vi "ReadSettings.vi"() -> (1 "Settings":T1)   [LabVIEW 2015]
uses:
  <vilib>/Utility/sysdir.llb/System Directory Type.ctl
  <vilib>/registry/registry.llb/Registry RtKey.ctl
  <vilib>/registry/registry.llb/Registry SAM.ctl
  Ctrls/YesOrNo.ctl
  <vilib>/Utility/config.llb/Read Key (U32).vi
  <vilib>/registry/registry.llb/Read Registry Value Simple STR.vi
  <vilib>/Utility/config.llb/Write Key (U32).vi
  <vilib>/Utility/config.llb/Read Key (Boolean).vi
  <vilib>/Utility/config.llb/Write Key (Boolean).vi
  <vilib>/Utility/config.llb/NI_LVConfig.lvlib
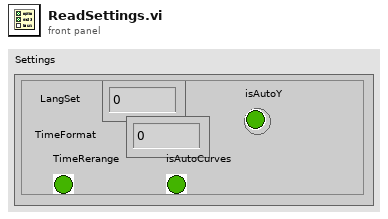
[diagram p1: front panel]
types:
  T1 = cluster{"LangSet":u32, "TimeFormat":u16, "TimeRerange":bool, "isAutoCurves":bool, "isAutoY":bool}
  T2 = typedef "System Directory Type.ctl" = i32
  T3 = typedef "NI_LVConfig.lvlib/Config Data RefNum.ctl" = refnum<k1>
  T4 = typedef "Registry SAM.ctl" = enum32{"KEY_QUERY_VALUE", "KEY_SET_VALUE", "KEY_CREATE_SUB_KEY", "KEY_ENUMERATE_SUB_KEYS", "KEY_NOTIFY", "KEY_CREATE_LINK", "KEY_READ", "KEY_WRITE", "KEY_ALL_ACCESS", "KEY_READ | KEY_WRITE"}
  T5 = typedef "Registry RtKey.ctl" = enum32{"HKEY_CLASSES_ROOT", "HKEY_CURRENT_USER", "HKEY_LOCAL_MACHINE", "HKEY_USERS", "HKEY_PERFORMANCE_DATA", "HKEY_CURRENT_CONFIG", "HKEY_DYN_DATA"}
  T6 = typedef "Registry refnum.ctl" = refnum<k1>
  T7 = typedef "YesOrNo.ctl" = bool
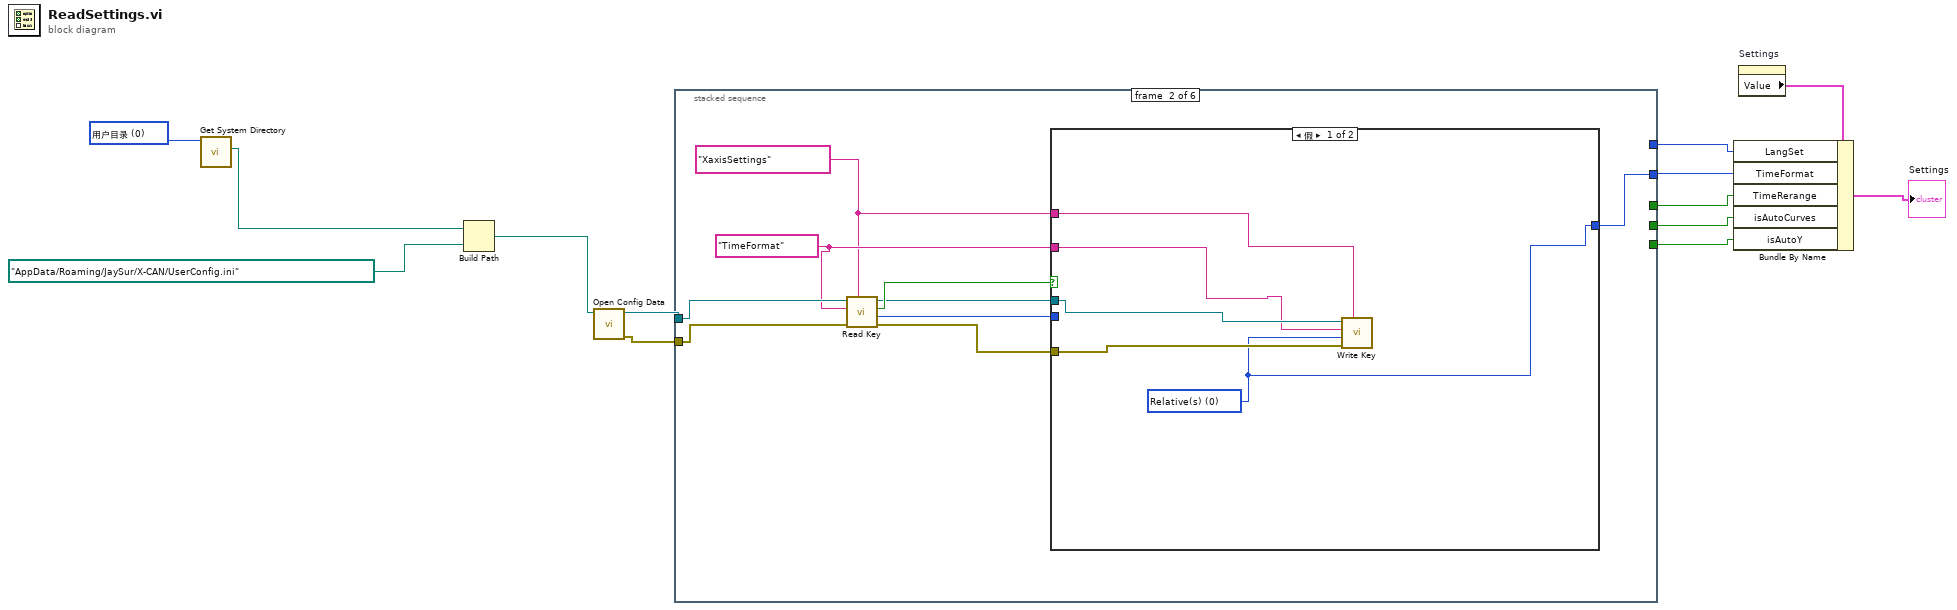
[diagram p0: block diagram]
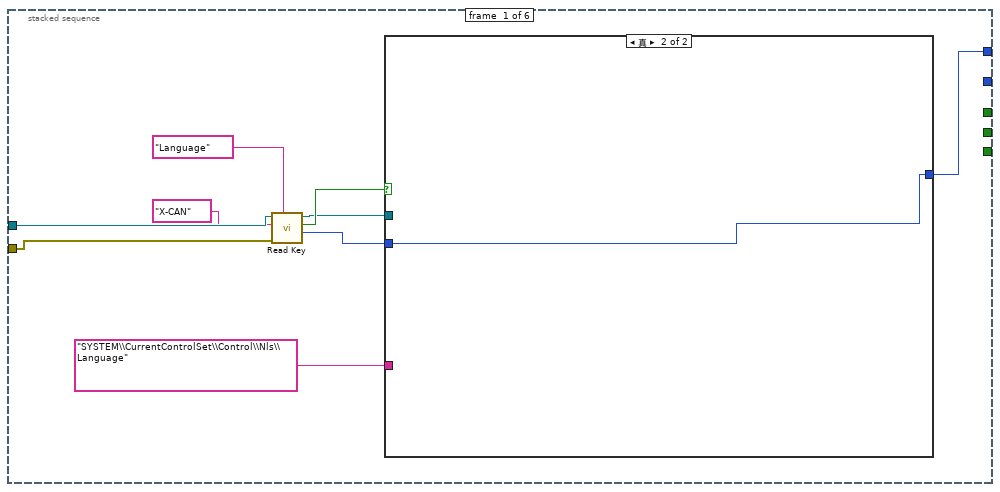
[diagram p2: hidden frame]
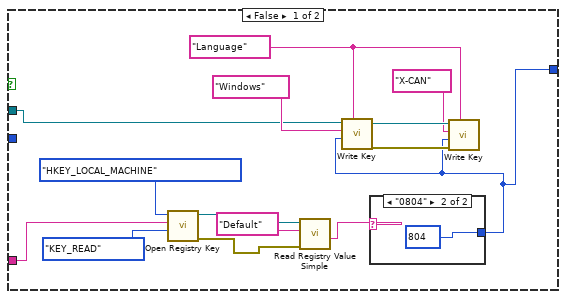
[diagram p3: hidden frame]
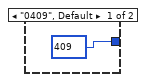
[diagram p4: hidden frame]
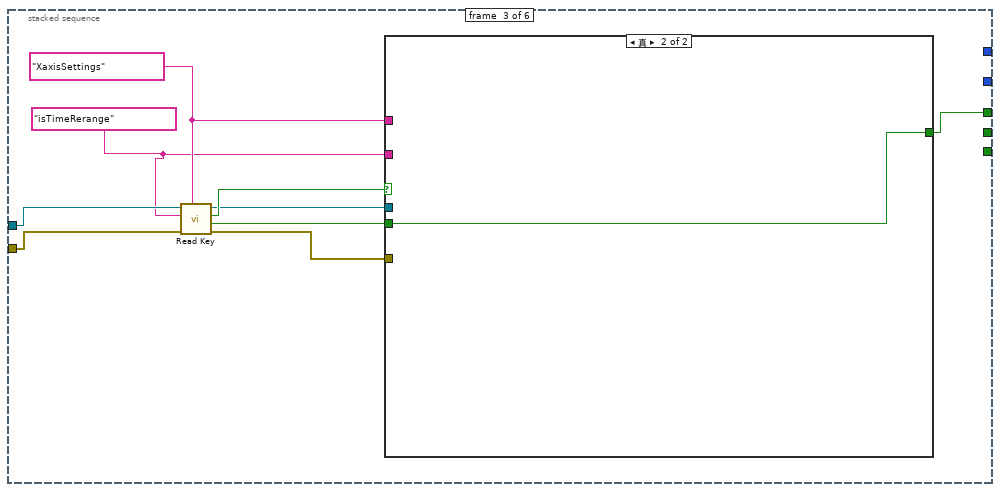
[diagram p6: hidden frame]
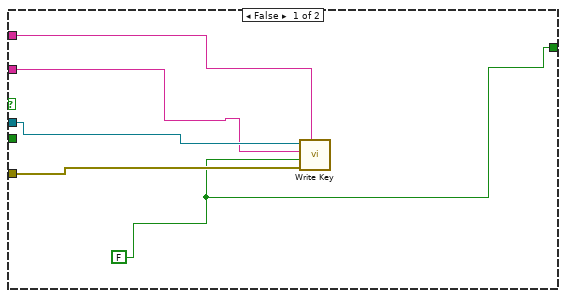
[diagram p7: hidden frame]
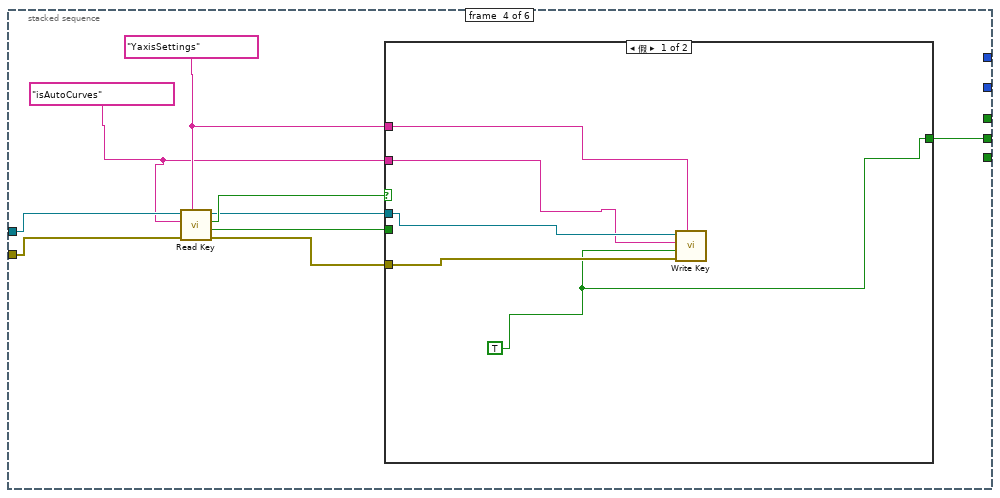
[diagram p8: hidden frame]
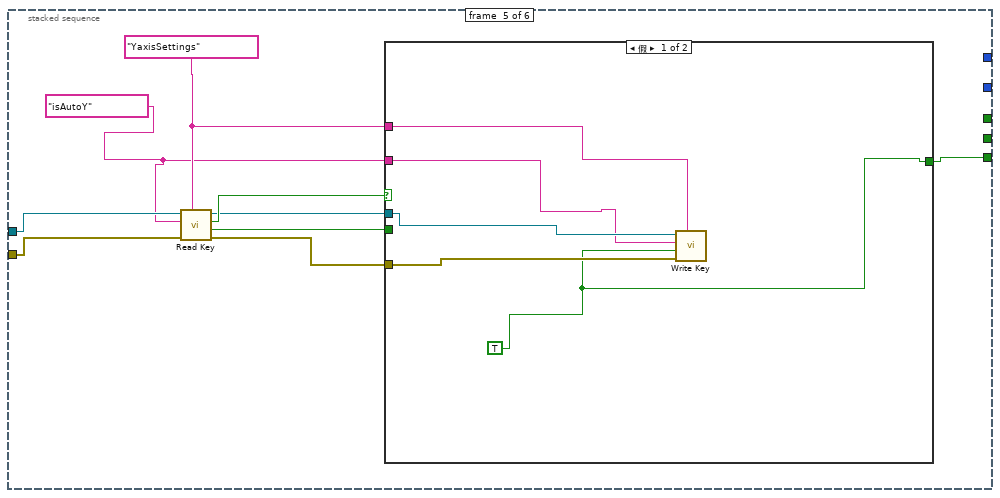
[diagram p10: hidden frame]
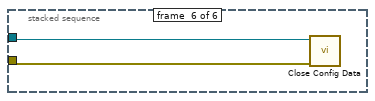
[diagram p12: hidden frame]
diagram:
  w12 = T2 0 items=["用户目录"=0, "用户桌面"=1, "用户文档"=2, "用户应用程序数据"=3, "用户设置"=4, "用户临时目录"=5, "公共文档"=6, "公共应用程序数据"=7, "公共设置"=8, "公共缓存"=13, "系统核心库"=9, "系统安装库"=10, "应用程序文件"=11, "启动盘根目录"=12] ("system directory type")
  n1 = call <vilib>:"Get System Directory.vi"("system directory type"=w12) -> ("system directory"=w11:path)  [unwired: 10 in]
  n2 = Build Path(base path=w11, name or relative path=path "AppData/Roaming/JaySur/X-CAN/UserConfig.ini" ("default name")) -> (appended path=w8:path)
  n3 = call <vilib>:"Open Config Data.vi"("configuration file path"=w8) -> ("error out"=w9:errorcluster, "refnum"=w10:T3)  [unwired: 8 in, 1 out]
  n4 = stacked-sequence {
    tunnel: w10 -> [w21 w48 w63 w78 w93 w101]
    tunnel: w9 -> [w18 w47 w62 w77 w92 w100]
    tunnel: [w14 _ _ _ _ _] -> w6
    tunnel: [_ w40 _ _ _ _] -> w5
    tunnel: [_ _ w55 _ _ _] -> w4
    tunnel: [_ _ _ w72 _ _] -> w3
    tunnel: [_ _ _ _ w86 _] -> w2
    frame #0 {
      n5 = call-poly <vilib>:"Read Key.vi"("section"="Language", "error in (no error)"=w18, "key"="X-CAN", "refnum"=w21) -> ("value"=w17:u32, "found?"=w19:bool, "refnum out"=w16:T3)  [unwired: 4 in, 1 out]
      n6 = case shown="真" w19 {
        tunnel: w17 -> [_ w39]
        tunnel: w16 -> [w25 _]
        tunnel: "SYSTEM\\CurrentControlSet\\Control\\Nls\\Language" ("subkey") -> [w24 _]
        tunnel: [w23 w39] -> w14
        frame False {
          w35 = "Language" ("section")
          n7 = call <vilib>:"Open Registry Key.vi"("security access mask (KEY_READ | KEY_WRITE)"=Registry_SAM."KEY_READ", "subkey"=w24, "root key (HKEY_LOCAL_MACHINE)"=Registry_RtKey."HKEY_LOCAL_MACHINE") -> ("error out"=w27:errorcluster, "refnum out"=w28:T6)  [unwired: 7 in]
          n8 = call-poly <vilib>:"Read Registry Value Simple.vi"("error in (no error)"=w27, "value"="Default", "refnum"=w28) -> ("String/Binary data"=w26:string)  [unwired: 3 in, 3 out]
          n9 = case shown="\"0804\"" w26 {
            tunnel: [u32 409 u32 804] -> w23
            frame "0409", Default {
            }
            frame "0804" {
            }
          }
          n10 = call-poly <vilib>:"Write Key.vi"("section"=w35, "value"=w23, "key"="Windows", "refnum"=w25) -> ("error out"=w36:errorcluster, "refnum out"=w33:T3)  [unwired: 5 in, 1 out]
          n11 = call-poly <vilib>:"Write Key.vi"("section"=w35, "error in (no error)"=w36, "value"=w23, "key"="X-CAN", "refnum"=w33) -> ()  [unwired: 4 in, 3 out]
        }
        frame True {
        }
      }
    }
    frame #1 {
      w42 = "XaxisSettings" ("section")
      w43 = "TimeFormat" ("key")
      n12 = call-poly <vilib>:"Read Key.vi"("section"=w42, "error in (no error)"=w47, "key"=w43, "refnum"=w48) -> ("error out"=w45:errorcluster, "value"=w41:u32, "found?"=w46:bool, "refnum out"=w44:T3)  [unwired: 4 in]
      n13 = case shown="假" w46 {
        tunnel: w45 -> [w53 _]
        tunnel: w44 -> [w52 _]
        tunnel: w43 -> [w51 _]
        tunnel: w42 -> [w50 _]
        tunnel: w41 -> [_ w54]
        tunnel: [w49 w54] -> w40
        frame False {
          w49 = u16 0 items=["Relative(s)", "Abs(noDate)", "Abs(withDate)"] ("TimeFormat")
          n14 = call-poly <vilib>:"Write Key.vi"("section"=w50, "error in (no error)"=w53, "value"=w49, "key"=w51, "refnum"=w52) -> ()  [unwired: 4 in, 3 out]
        }
        frame True {
        }
      }
    }
    frame #2 {
      w56 = "isTimeRerange" ("key")
      w58 = "XaxisSettings" ("section")
      n15 = call-poly <vilib>:"Read Key.vi"("section"=w58, "error in (no error)"=w62, "key"=w56, "refnum"=w63) -> ("error out"=w60:errorcluster, "value"=w57:bool, "found?"=w61:bool, "refnum out"=w59:T3)  [unwired: 4 in]
      n16 = case shown="真" w61 {
        tunnel: w60 -> [w68 _]
        tunnel: w59 -> [w67 _]
        tunnel: w56 -> [w66 _]
        tunnel: w58 -> [w65 _]
        tunnel: w57 -> [_ w69]
        tunnel: [w64 w69] -> w55
        frame False {
          w64 = T7 FALSE ("isTimeRerange")
          n17 = call-poly <vilib>:"Write Key.vi"("section"=w65, "error in (no error)"=w68, "value"=w64, "key"=w66, "refnum"=w67) -> ()  [unwired: 4 in, 3 out]
        }
        frame True {
        }
      }
    }
    frame #3 {
      w70 = "isAutoCurves" ("key")
      w71 = "YaxisSettings" ("section")
      n18 = call-poly <vilib>:"Read Key.vi"("section"=w71, "error in (no error)"=w77, "key"=w70, "refnum"=w78) -> ("error out"=w75:errorcluster, "value"=w73:bool, "found?"=w76:bool, "refnum out"=w74:T3)  [unwired: 4 in]
      n19 = case shown="假" w76 {
        tunnel: w75 -> [w83 _]
        tunnel: w74 -> [w82 _]
        tunnel: w70 -> [w81 _]
        tunnel: w71 -> [w80 _]
        tunnel: w73 -> [_ w84]
        tunnel: [w79 w84] -> w72
        frame False {
          w79 = T7 TRUE ("isTimeRerange")
          n20 = call-poly <vilib>:"Write Key.vi"("section"=w80, "error in (no error)"=w83, "value"=w79, "key"=w81, "refnum"=w82) -> ()  [unwired: 4 in, 3 out]
        }
        frame True {
        }
      }
    }
    frame #4 {
      w85 = "isAutoY" ("key")
      w87 = "YaxisSettings" ("section")
      n21 = call-poly <vilib>:"Read Key.vi"("section"=w87, "error in (no error)"=w92, "key"=w85, "refnum"=w93) -> ("error out"=w90:errorcluster, "value"=w88:bool, "found?"=w91:bool, "refnum out"=w89:T3)  [unwired: 4 in]
      n22 = case shown="假" w91 {
        tunnel: w90 -> [w98 _]
        tunnel: w89 -> [w97 _]
        tunnel: w85 -> [w96 _]
        tunnel: w87 -> [w95 _]
        tunnel: w88 -> [_ w99]
        tunnel: [w94 w99] -> w86
        frame False {
          w94 = T7 TRUE ("isTimeRerange")
          n23 = call-poly <vilib>:"Write Key.vi"("section"=w95, "error in (no error)"=w98, "value"=w94, "key"=w96, "refnum"=w97) -> ()  [unwired: 4 in, 3 out]
        }
        frame True {
        }
      }
    }
    frame #5 {
      n24 = call <vilib>:"Close Config Data.vi"("error in (no error)"=w100, "refnum"=w101) -> ()  [unwired: 8 in, 2 out]
    }
  }
  n25 = property on="Settings" class="Clust (严格)"() -> ("Value"=w7:T1)  [unwired: 2 in, 2 out]
  n26 = Bundle By Name(cluster=w7, "LangSet"=w6, "TimeFormat"=w5, "TimeRerange"=w4, "isAutoCurves"=w3, "isAutoY"=w2) -> (→"Settings":T1)
